vi "Voltage calculator.vi"(0 "ROT FL":string="My AI RefNum", 1 "ROT FR":string="My AI RefNum", 4 "ROT BL":string="My AI RefNum", 5 "ROT BR":string="My AI RefNum") -> (10 "Max FL":dbl, 11 "Max BL":dbl, 12 "Min FL":dbl, 13 "Min BL":dbl, 14 "Min FR":dbl, 15 "Max FR":dbl, 18 "Min BR":dbl, 19 "Max BR":dbl)   [LabVIEW 2014]
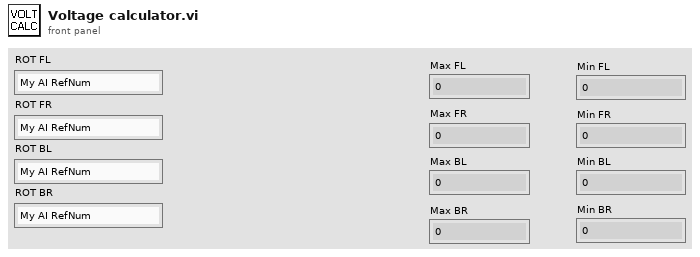
[diagram p1: front panel]
types:
  T1 = typedef "WPI_AnalogChannelDevRef.ctl" = cluster{"DevStatus":errorcluster, "Controller":T2, "Analog Channel":T3}
  T2 = typedef "FPGA_TypedefAnalogModule.ctl" = enum16{"Controller 1"}
  T3 = typedef "FPGA_AIChannel.ctl" = enum8{"AI 0", "AI 1", "AI 2", "AI 3", "AI MXP 0", "AI MXP 1", "AI MXP 2", "AI MXP 3", "Invalid"}
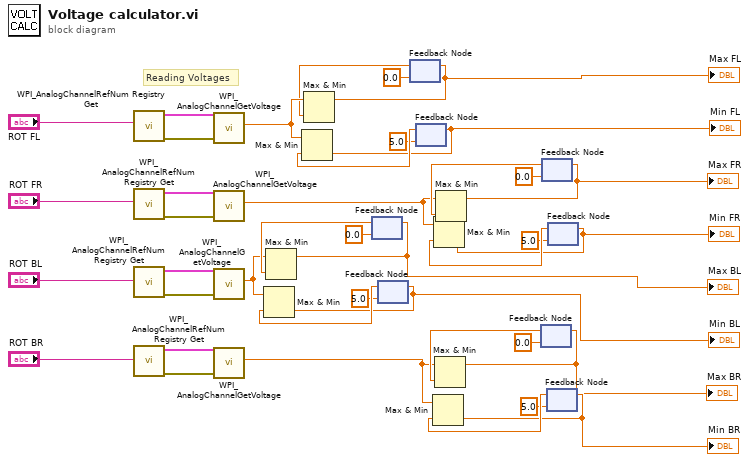
[diagram p0: block diagram]
diagram:
  # "Reading Voltages"
  n1 = call <vilib>:"WPI_AnalogChannelRefNum Registry Get.vi"("refnum name"="ROT FL") -> ("error out"=w39:errorcluster, "AIDeviceRef"=w40:T1)  [unwired: 9 in]
  n2 = call <vilib>:"WPI_AnalogChannelRefNum Registry Get.vi"("refnum name"="ROT FR") -> ("error out"=w37:errorcluster, "AIDeviceRef"=w38:T1)  [unwired: 9 in]
  n3 = call <vilib>:"WPI_AnalogChannelRefNum Registry Get.vi"("refnum name"="ROT BL") -> ("error out"=w1:errorcluster, "AIDeviceRef"=w36:T1)  [unwired: 9 in]
  n4 = call <vilib>:"WPI_AnalogChannelRefNum Registry Get.vi"("refnum name"="ROT BR") -> ("error out"=w34:errorcluster, "AIDeviceRef"=w35:T1)  [unwired: 9 in]
  n5 = call <vilib>:"WPI_AnalogChannelGetVoltage.vi"("error in (no error)"=w39, "AIDeviceRef"=w40) -> ("Voltage"=w29:dbl)  [unwired: 7 in, 2 out]
  n6 = call <vilib>:"WPI_AnalogChannelGetVoltage.vi"("error in (no error)"=w37, "AIDeviceRef"=w38) -> ("Voltage"=w12:dbl)  [unwired: 7 in, 2 out]
  n7 = call <vilib>:"WPI_AnalogChannelGetVoltage.vi"("error in (no error)"=w1, "AIDeviceRef"=w36) -> ("Voltage"=w11:dbl)  [unwired: 7 in, 2 out]
  n8 = call <vilib>:"WPI_AnalogChannelGetVoltage.vi"("error in (no error)"=w34, "AIDeviceRef"=w35) -> ("Voltage"=w10:dbl)  [unwired: 7 in, 2 out]
  n9 = feedback #1(0.0) -> (w19:dbl)
  n10 = Max & Min(x=w11, y=w19) -> (max(x,y)=w5:dbl)  [unwired: 1 out]
  "Max BL" <- w5
  n11 = feedback-in #1(w5) -> ()
  n12 = feedback #2(5.0) -> (w20:dbl)
  n13 = Max & Min(x=w11, y=w20) -> (min(x,y)=w4:dbl)  [unwired: 1 out]
  "Min BL" <- w4
  n14 = feedback-in #2(w4) -> ()
  n15 = feedback #3(0.0) -> (w27:dbl)
  n16 = Max & Min(x=w29, y=w27) -> (max(x,y)=w9:dbl)  [unwired: 1 out]
  "Max FL" <- w9
  n17 = feedback-in #3(w9) -> ()
  n18 = feedback #4(5.0) -> (w28:dbl)
  n19 = Max & Min(x=w29, y=w28) -> (min(x,y)=w8:dbl)  [unwired: 1 out]
  "Min FL" <- w8
  n20 = feedback-in #4(w8) -> ()
  n21 = feedback #5(0.0) -> (w15:dbl)
  n22 = Max & Min(x=w10, y=w15) -> (max(x,y)=w2:dbl)  [unwired: 1 out]
  "Max BR" <- w2
  n23 = feedback-in #5(w2) -> ()
  n24 = feedback #6(0.0) -> (w23:dbl)
  n25 = Max & Min(x=w12, y=w23) -> (max(x,y)=w7:dbl)  [unwired: 1 out]
  "Max FR" <- w7
  n26 = feedback-in #6(w7) -> ()
  n27 = feedback #7(5.0) -> (w16:dbl)
  n28 = Max & Min(x=w10, y=w16) -> (min(x,y)=w3:dbl)  [unwired: 1 out]
  "Min BR" <- w3
  n29 = feedback-in #7(w3) -> ()
  n30 = feedback #8(5.0) -> (w24:dbl)
  n31 = Max & Min(x=w12, y=w24) -> (min(x,y)=w6:dbl)  [unwired: 1 out]
  "Min FR" <- w6
  n32 = feedback-in #8(w6) -> ()
